vi "Text Description.vi"(11 "Message":refnum<class "Observer_RegisterByLabel.lvclass">) -> (2 "Description":string, 3 "Message":refnum<class "Observer_RegisterByLabel.lvclass">)   [LabVIEW 2011, in "Messenging.lvlib" / "Observer_RegisterByLabel.lvclass"]
uses:
  Observer_RegisterByLabel.lvclass
  ParentCommand/ObserverRegistryCommand.lvclass
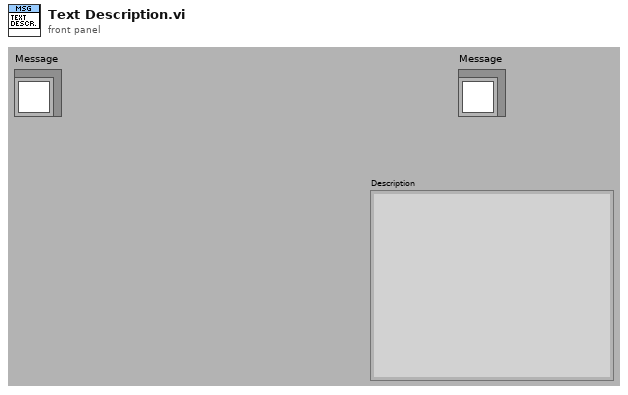
[diagram p1: front panel]
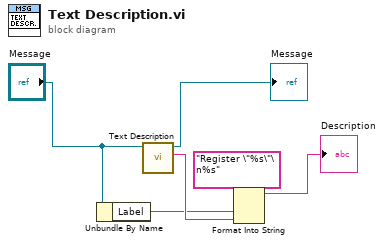
[diagram p0: block diagram]
diagram:
  n1 = Unbundle By Name("Message") -> ("Label"=w2:string)
  n2 = call-parent "Text Description.vi"("Message"="Message") -> ("Description"=w3:string, "Message"=→"Message":refnum<class "Observer_RegisterByLabel.lvclass">)  [unwired: 9 out]
  n3 = Format Into String(format string="Register \"%s\"\n%s", w2, w3) -> (resulting string=→"Description":string)  [unwired: 2 in, 1 out]
